vi "Read Dispenser Hardware Path.vi"(8 "error in":errorcluster, 11 "Config Manager in":refnum<class "Config Manager Class.lvclass">) -> (0 "error out":errorcluster, 2 "Hardware Path":string, 3 "Config Manager out":refnum<class "Config Manager Class.lvclass">)   [LabVIEW 2011, in "Config Manager Class.lvclass"]
uses:
  Config Manager Class.lvclass
  Config Manager Class.lvclass/Config Manager Class.ctl
  <vilib>/Utility/config.llb/Read Key (String).vi
  <vilib>/Utility/config.llb/NI_LVConfig.lvlib
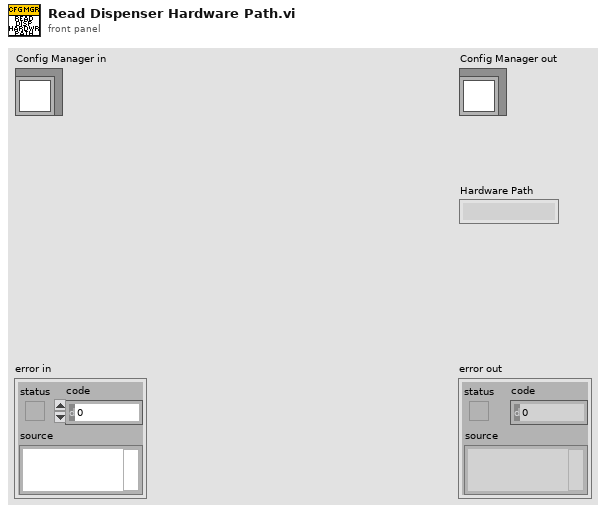
[diagram p1: front panel]
types:
  T1 = typedef "NI_LVConfig.lvlib/Config Data RefNum.ctl" = refnum<k1>
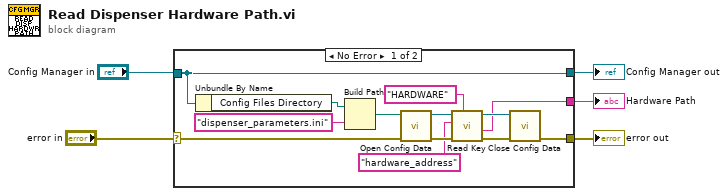
[diagram p0: block diagram]
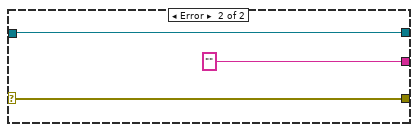
[diagram p2: hidden frame]
diagram:
  n1 = case shown="No Error" "error in" {
    selector: "error in" -> [w18 w21]
    tunnel: [w7 w21] -> w1
    tunnel: [w9 w19] -> w2
    tunnel: "Config Manager in" -> [w9 w19]
    tunnel: [w8 "" ("value")] -> w3
    frame No Error {
      n2 = Unbundle By Name(w9) -> ("Config Files Directory"=w10:path)
      n3 = Build Path(base path=w10, name or relative path="dispenser_parameters.ini") -> (appended path=w6:path)
      n4 = call <vilib>:"Open Config Data.vi"("error in (no error)"=w18, "configuration file path"=w6) -> ("error out"=w13:errorcluster, "refnum"=w15:T1)  [unwired: 7 in, 1 out]
      n5 = call-poly <vilib>:"Read Key.vi"("section"="HARDWARE", "error in (no error)"=w13, "key"="hardware_address" ("format string"), "refnum"=w15) -> ("error out"=w16:errorcluster, "value"=w8:string, "refnum out"=w17:T1)  [unwired: 4 in, 1 out]
      n6 = call <vilib>:"Close Config Data.vi"("error in (no error)"=w16, "refnum"=w17) -> ("error out"=w7:errorcluster)  [unwired: 8 in, 1 out]
    }
    frame Error {
    }
  }
  "error out" <- w1
  "Config Manager out" <- w2
  "Hardware Path" <- w3
